vi "Send Number Of Neopixels.vi"(8 "Error In":errorcluster, 11 "Display In":refnum<class "Display.lvclass">) -> (0 "Error Out":errorcluster, 3 "Display Out":refnum<class "Display.lvclass">)   [LabVIEW 2019, in "Display.lvclass"]
uses:
  Display.lvclass
  Shared/Public/Controls/Neopixel FIFO Command.ctl
  Shared/Neopixel Shared.lvlib
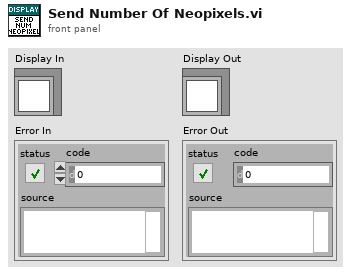
[diagram p1: front panel]
types:
  T1 = typedef "Neopixel Shared.lvlib/Neopixel FIFO Command.ctl" = enum8{"Set Number Of Neopixels", "Update Frame"}
  T2 = typedef "Display.lvclass/Size.ctl" = cluster{"Width":i32, "Height":i32}
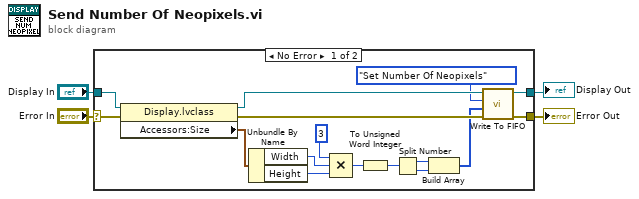
[diagram p0: block diagram]
diagram:
  n1 = case shown="No Error" "Error In" {
    selector: "Error In" -> [w17 w21]
    tunnel: "Display In" -> [w18 w22]
    tunnel: [w16 w21] -> w2
    tunnel: [w15 w22] -> w1
    frame No Error {
      n2 = property class="Display.lvclass"(reference=w18, error in=w17) -> (reference out=w19:refnum<class "Display.lvclass">, error out=w20:errorcluster, "Accessors:Size"=w5:T2)
      n3 = Unbundle By Name(w5) -> ("Width"=w6:i32, "Height"=w7:i32)
      n4 = Compound Arithmetic op=MULTIPLY(3 ("value"), w6, w7) -> (w11:i32)
      n5 = To Unsigned Word Integer(number=w11) -> (unsigned 16bit integer=w12:u16)
      n6 = Split Number(x=w12) -> (hi(x)=w13:u8, lo(x)=w14:u8)
      n7 = Build Array(w13, w14) -> (w10:u8[])
      n8 = call "Write To FIFO.vi"("Error In"=w20, "Data"=w10, "Command"=Neopixel_FIFO_Command."Set Number Of Neopixels", "Display In"=w19) -> ("Error Out"=w16:errorcluster, "Display Out"=w15:refnum<class "Display.lvclass">)  [unwired: 6 in]
    }
    frame Error {
    }
  }
  "Error Out" <- w2
  "Display Out" <- w1
